vi "set_params.vi"(8 "error in (no error)":errorcluster caption="entrée d'erreur (pas d'erreur)", 11 "BaggingRegressor.lvclass":refnum<class "BaggingRegressor.lvclass">) -> (0 "error out":errorcluster caption="sortie d'erreur", 3 "BaggingRegressor.lvclass 2":refnum<class "BaggingRegressor.lvclass">)   [LabVIEW 2020, in "BaggingRegressor.lvclass"]
uses:
  BaggingRegressor.lvclass
  BaggingRegressor.lvclass/BaggingRegressor.ctl
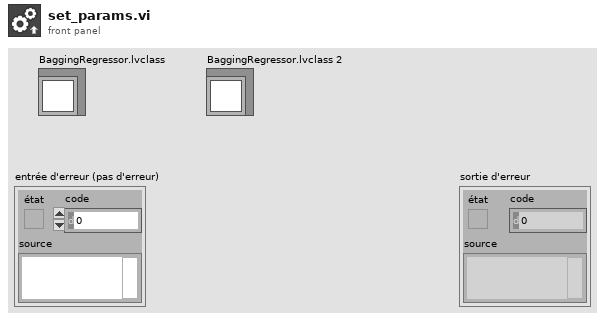
[diagram p1: front panel]
types:
  T1 = typedef "bagging_regressor_params.ctl" = cluster{"base_estimator":string, "n_estimators":dbl, "max_samples":cluster{"max_samples_type":string, "max_samples_float":dbl, "max_samples_int":dbl}, "max_features":cluster{"max_features_type":string, "max_features_float":dbl, "max_features_int":dbl}, "bootstrap":bool, "bootstrap_features":bool, "oob_score":bool, "warm_start":bool, "n_jobs":dbl, "random_state":dbl, "verbose":dbl}
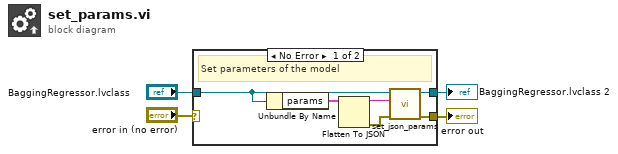
[diagram p0: block diagram]
diagram:
  n1 = case shown="No Error" "error in (no error)" {
    selector: "error in (no error)" -> [_ w12]
    tunnel: [w7 w12] -> w3
    tunnel: [w8 w11] -> w1
    tunnel: "BaggingRegressor.lvclass" -> [w5 w11]
    frame No Error {
      # "Set parameters of the model"
      n2 = Unbundle By Name(w5) -> ("params"=w10:T1)
      n3 = Flatten To JSON(anything=w10) -> (JSON string=w9:string, 11:w6:errorcluster)  [unwired: 2 in]
      n4 = call-dynamic "set_json_params.vi"("error in (no error)"=w6, "params"=w9, "Model en entrée"=w5) -> ("error out"=w7:errorcluster, "Model en sortie"=w8:refnum<class "BaggingRegressor.lvclass">)  [unwired: 7 in]
    }
    frame Error {
    }
  }
  "error out" <- w3
  "BaggingRegressor.lvclass 2" <- w1
